vi "Value Set.vi"(7 "Value Set":u16(ring) items=["Input Selection"=2000, "Status"=2010, "Set Current"=2020, "Set Voltage"=2021, "Current Limitation"=2030, "Voltage Limitation"=2031, "Current Error Threshold"=2032, "Voltage Error Threshold"=2033, "Channel Baud Rate"=2050, "Response Delay"=2052, "Timeout"=2060, "Target Object Temperature"=3000, "Coarse Temp Ramp"=3003, "Proximity Width"=3002, "Kp"=3010, "Ti"=3011, "Td"=3012, "D Part Damping D1"=3013, "Live Enable"=50000, "Live Set Current"=50001, "Live Set Voltage"=50002, "Object Target Temperature"=50012, "Save Data to Flash"=108], 8 "Value":string="01", 9 "Sequence":string="0000", 10 "Instance":string="01", 11 "TEC 1090":refnum<class "Meerstetter TEC.lvclass">) -> (2 "hex integer string":string, 3 "TEC 1091":refnum<class "Meerstetter TEC.lvclass">)   [LabVIEW 2014, in "Meerstetter TEC.lvclass"]
uses:
  Meerstetter TEC.lvclass
  Meerstetter TEC.lvclass/Meerstetter TEC.ctl
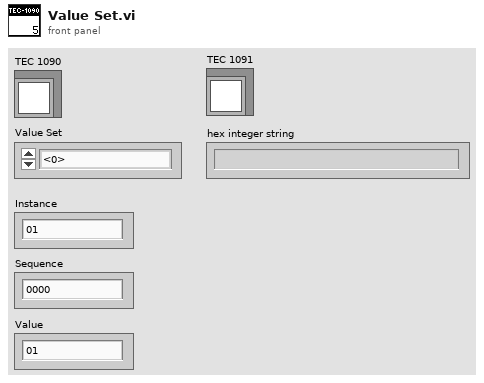
[diagram p1: front panel]
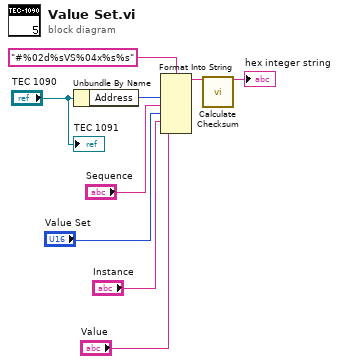
[diagram p0: block diagram]
diagram:
  n1 = Unbundle By Name("TEC 1090") -> ("Address"=w3:u8)
  n2 = Format Into String(format string="#%02d%sVS%04x%s%s", w3, "Sequence", "Value Set", "Instance", "Value") -> (resulting string=w6:string)  [unwired: 2 in, 1 out]
  n3 = call "Calculate Checksum.vi"("Message"=w6) -> ("MSG"=→"hex integer string":string)  [unwired: 11 in, 3 out]
  "TEC 1091" <- "TEC 1090"
